vi "XGT 개별쓰기 Enquire.vi"(5 "명령어타입":string="SS", 7 "명령어":string="W", 9 "블록 데이터":T1(array[cluster])=[{"변수길이"="06", "변수이름"="%MW230", "데이터"="00FF"}], 10 "블록수":string="01", 11 "국번":string="01") -> (3 "연속연결 Enquire문":string)   [LabVIEW 2012]
panel:
  in  "Header":string="\u0005"
  in  "BCC":string
  in  "Tail":string="\u0004"
  # "국번 1의 M230 번지에 헥사 FF를 쓸 경우"
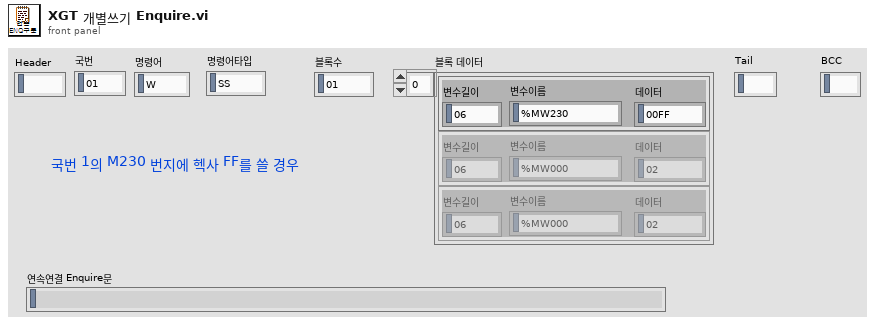
[diagram p1: front panel]
types:
  T1 = cluster{"변수길이":string, "변수이름":string, "데이터":string}[]
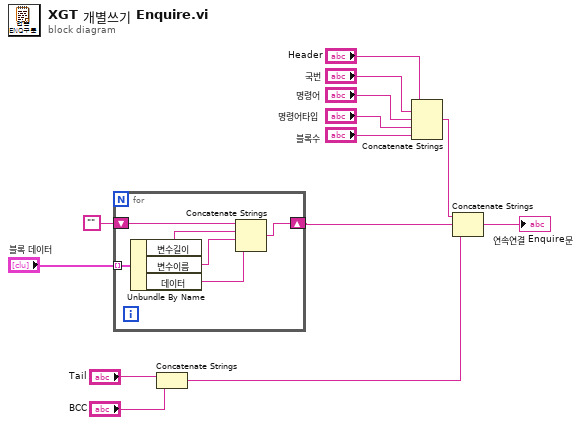
[diagram p0: block diagram]
diagram:
  n1 = for {
    tunnel: "블록 데이터" -> [w19] mode=indexing
    shift-right: [w14] -> w3
    shift-left: "" -> [w18]
    n2 = Unbundle By Name(w19) -> ("변수길이"=w17:string, "변수이름"=w16:string, "데이터"=w15:string)
    n3 = Concatenate Strings(w18, w17, w16, w15) -> (w14:string)
  }
  n4 = Concatenate Strings("Tail", "BCC") -> (w2:string)
  n5 = Concatenate Strings("Header", "국번", "명령어", "명령어타입", "블록수") -> (w4:string)
  n6 = Concatenate Strings(w4, w3, w2) -> (→"연속연결 Enquire문":string)
